vi "ExpInvokeMethod.vi"(0 "ExpID":string, 1 "Method Name":string, 2 "Argument(s)":variant, 3 "Rsp. Type (or value to update)":variant, 4 "Require Response":bool, 5 "error in (no error)":errorcluster) -> (14 "ExpID out":string, 15 "Response":variant, 19 "error out":errorcluster)   [LabVIEW 2017]
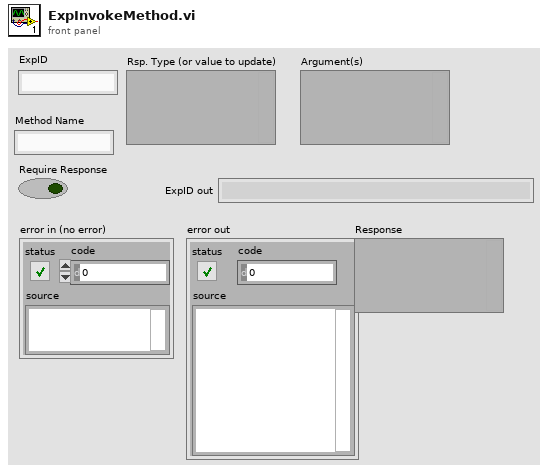
[diagram p1: front panel]
types:
  T1 = typedef "ExperimentInfo.ctl" = cluster{"ExposeInfo":T2, "ExpID":string, "ExperimentFilename":string, "Caller Keep Alive":refnum<data-value>}
  T2 = typedef "ExposeInfo.ctl" = cluster{"CSCom":refnum<k24>, "URL":string, "Events Category":string, "ID":string, "SRefID":string}
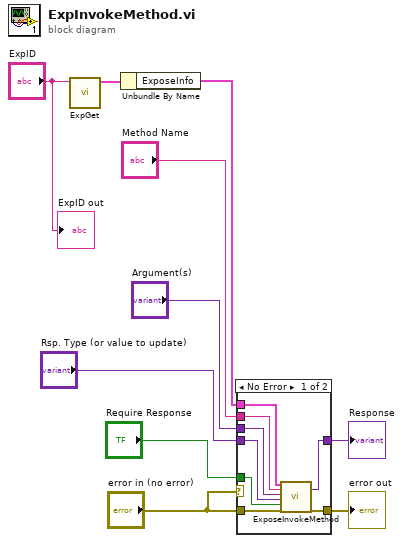
[diagram p0: block diagram]
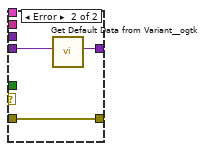
[diagram p2: hidden frame]
diagram:
  n1 = call "ExpGet.vi"("ExpID"="ExpID") -> ("Exp Info"=w5:T1)  [unwired: 9 in, 1 out]
  n2 = Unbundle By Name(w5) -> ("ExposeInfo"=w4:T2)
  n3 = case shown="No Error" "error in (no error)" {
    tunnel: "Method Name" -> [w18 _]
    tunnel: "Argument(s)" -> [w17 _]
    tunnel: "Require Response" -> [w16 _]
    tunnel: "error in (no error)" -> [w15 w21]
    tunnel: [w14 w21] -> w7
    tunnel: w4 -> [w13 _]
    tunnel: "Rsp. Type (or value to update)" -> [w12 w20]
    tunnel: [w11 w19] -> w1
    frame No Error {
      n4 = call "ExposeInvokeMethod.vi"("Expose Info in"=w13, "Method Name"=w18, "Argument(s)"=w17, "Rsp. Type (or value to update)"=w12, "Require Response"=w16, "error in (no error)"=w15) -> ("Response"=w11:variant, "error out"=w14:errorcluster)  [unwired: 11 in, 1 out]
    }
    frame Error {
      n5 = call <userlib>:"Get Default Data from Variant__ogtk.vi"("Variant"=w20) -> ("Default VData"=w19:variant)  [unwired: 9 in, 1 out]
    }
  }
  "error out" <- w7
  "Response" <- w1
  "ExpID out" <- "ExpID"
